vi "RG DAQ control for PIA.vi"(8 "error in":errorcluster, 10 "lines":string="Dev1/port1/line0", 11 "Initial value":bool) -> ()   [LabVIEW 2015]
uses:
  <vilib>/DAQmx/write.llb/DAQmx Write.vi
  <vilib>/DAQmx/write.llb/DAQmx Write (Digital 1D Bool NChan 1Samp 1Line).vi
  <vilib>/DAQmx/create/channels.llb/DAQmx Create Channel (DO-Digital Output).vi
  <vilib>/DAQmx/miscellaneous.llb/DAQmx Fill In Error Info.vi
  <resource>/objmgr/daqmx.rc
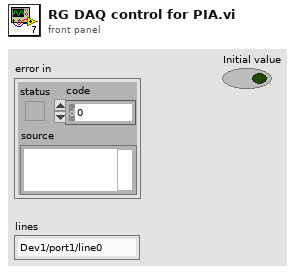
[diagram p1: front panel]
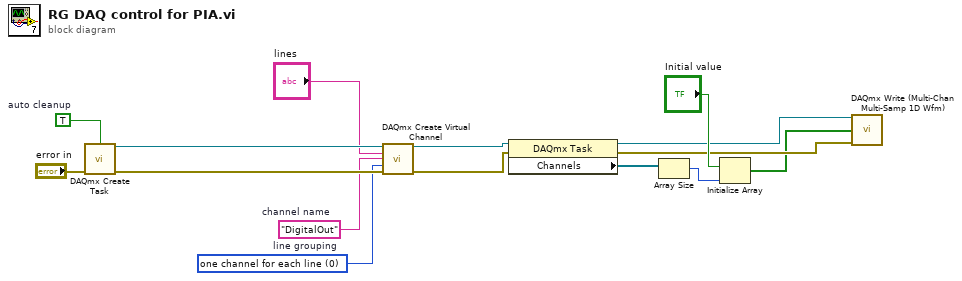
[diagram p0: block diagram]
diagram:
  w10 = 0 items=["one channel for each line", "one channel for all lines"]  # line grouping
  w9 = "DigitalOut"  # channel name
  w13 = TRUE  # auto cleanup
  n1 = call <vilib>:"DAQmx Create Task.vi"("auto cleanup"=w13, "error in"="error in") -> ("task out"=w12:refnum<k21>, "error out"=w14:errorcluster)  [unwired: 12 in]
  n2 = call-poly <vilib>:"DAQmx Create Virtual Channel.vi"("task in"=w12, "lines"="lines", "name to assign"=w9, "line grouping"=w10, "error in"=w14) -> ("task out"=w6:refnum<k21>, "error out"=w5:errorcluster)  [unwired: 9 in]
  n3 = property class="DAQmx Task"(reference=w6, error in=w5) -> (reference out=w3:refnum<k21>, error out=w2:errorcluster, "Channels"=w8:refnum<k21>[])
  n4 = Array Size(array=w8) -> (size(s)=w7:i32)
  n5 = Initialize Array("Initial value", w7) -> (w1:bool[])
  n6 = call-poly "DAQmx Write (Multi-Chan Multi-Samp 1D Wfm).vi"("task/channels in"=w3, "data"=w1, "error in"=w2) -> ()  [unwired: 10 in, 3 out]
